vi "DeviceStop.vi"(7 "error in":errorcluster, 11 "Handle In":u64[](array[numeric])) -> (2 "Result":i32, 3 "Handle Out":u64[](array[numeric]), 5 "error out":errorcluster)   [LabVIEW 2020, in "SnapMB.lvlib"]
uses:
  SnapMB.lvlib
  windows/snapmb.dll
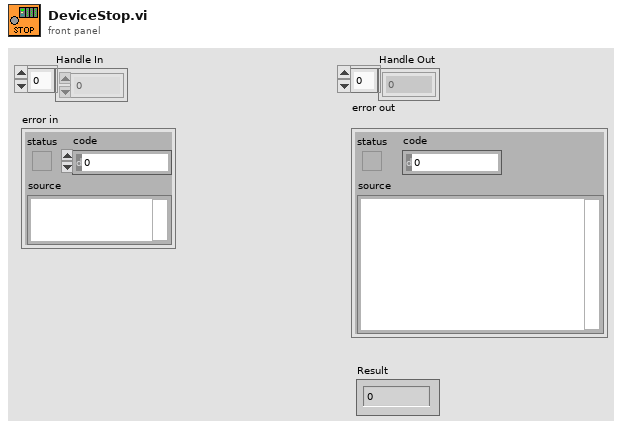
[diagram p1: front panel]
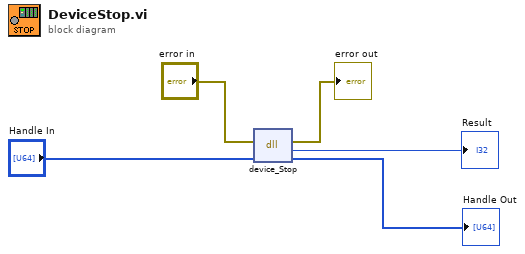
[diagram p0: block diagram]
diagram:
  n1 = dll-call lib="D:/SnapMB/LabView/lib/windows/snapmb.dll" fn="device_Stop"(error in="error in", "Device"="Handle In") -> (error out=→"error out":errorcluster, "Result"=→"Result":i32, "Device"=→"Handle Out":u64[])  [unwired: 2 in, 1 out]
